vi "PH_PSDBWriter.ProcEvents.vi"(0 "i ref in":refnum<vi>, 5 "error in":errorcluster) -> (14 "i ref out":refnum<vi>, 19 "error out":errorcluster)   [LabVIEW 2014, in "PH_PSDBWriter.lvlib"]
doc: "This method is used to define the events the object will listen to. Add your own events here."
uses:
  PH_PSDBWriter.lvlib
  CSCore/BaseProcess/BaseProcess.lvlib
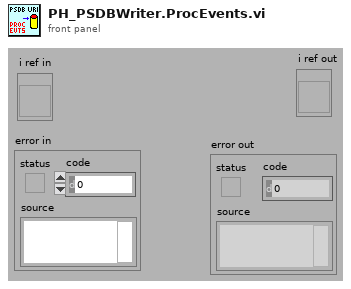
[diagram p1: front panel]
types:
  T1 = typedef "BaseProcess.lvlib/BaseProcess.event definition.ctl" = cluster{"CAEEvtDef":T2, "Data Descriptor":T3}
  T2 = typedef "CAEObj.lvlib/CAEObj.event definition.ctl" = cluster{"URL":string, "enable":bool, "ignoreResID":bool}
  T3 = typedef "BaseProcess.lvlib/BaseProcess.descriptor string definition.ctl" = string
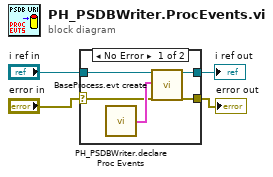
[diagram p0: block diagram]
diagram:
  n1 = case shown="No Error" "error in" {
    selector: "error in" -> [w5 w11]
    tunnel: "i ref in" -> [w6 w10]
    tunnel: [w9 w11] -> w3
    tunnel: [w8 w10] -> w2
    frame No Error {
      n2 = call "PH_PSDBWriter.declare Proc Events.vi"() -> ("PSDB DIM Service Events"=w7:T1[])  [unwired: 1 in]
      n3 = call "BaseProcess.evt create.vi"("i ref in"=w6, "newEvents"=w7, "error in (no error)"=w5) -> ("i ref out"=w8:refnum<vi>, "error out"=w9:errorcluster)  [unwired: 13 in, 2 out]
    }
    frame Error {
    }
  }
  "i ref out" <- w2
  "error out" <- w3
